vi "WAVeform_FORMat.vi"(7 "Write?":bool, 8 "Error":errorcluster, 11 "VISA resource name":refnum<visa-resource-name>) -> (0 "Error out":errorcluster, 2 "Format out":string, 3 "VISA resource name out":refnum<visa-resource-name>)   [LabVIEW 2020]
doc: "数据格式"
panel:
  out "读取缓冲区":string
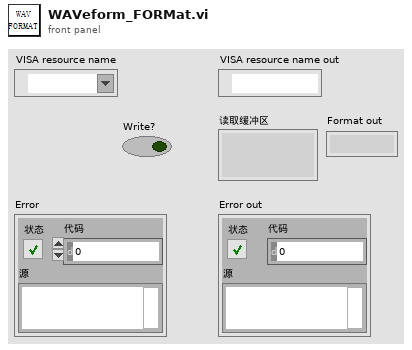
[diagram p1: front panel]
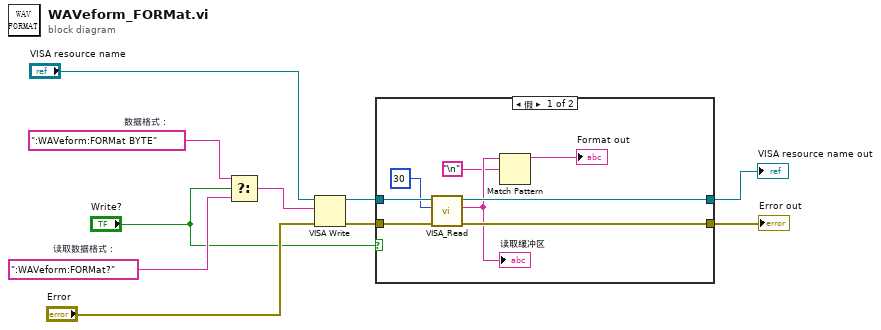
[diagram p0: block diagram]
diagram:
  w9 = ":WAVeform:FORMat?"  # 读取数据格式：
  w1 = ":WAVeform:FORMat BYTE"  # 数据格式：
  n1 = Select(t=w1, s="Write?", f=w9) -> (s? t:f=w8:string)
  n2 = VISA Write(VISA resource name="VISA resource name", write buffer=w8, error in (no error)="Error") -> (VISA resource name out=w4:refnum<visa-resource-name>, error out=w6:errorcluster)  [unwired: 1 out]
  n3 = case shown="假" "Write?" {
    tunnel: w4 -> [w18 w20]
    tunnel: w6 -> [w17 w19]
    tunnel: [w15 w19] -> w5
    tunnel: [w16 w20] -> w2
    frame False {
      n4 = call "VISA_Read.vi"("Error"=w17, "字节总数"=u32 30, "VISA resource name"=w18) -> ("Error out"=w15:errorcluster, "读取缓冲区"=w14:string, "VISA resource name out"=w16:refnum<visa-resource-name>)  [unwired: 6 in]
      "读取缓冲区" <- w14
      n5 = Match Pattern(string=w14, regular expression="\n") -> (before substring=→"Format out":string)  [unwired: 1 in, 3 out]
    }
    frame True {
    }
  }
  "VISA resource name out" <- w2
  "Error out" <- w5
